vi "PreCompileMainSeq.vi"(6 "steps":i32, 8 "error in (no error)":errorcluster, 9 "first seq":T1, 10 "Compiler Settings":T3={"Python Path"=path "", "Main File"="", "Meta File"="", "Aux File"="", "Pre File"="metascript.txt"}, 11 "queue in":refnum<queue>) -> (0 "error out":errorcluster)   [LabVIEW 2019]
uses:
  PulseCompiler/CompilerSettings.ctl
  Controller/PulseControl.ctl
  Params.ctl
  controls/GlobalExp.vi
  Global.lvlib
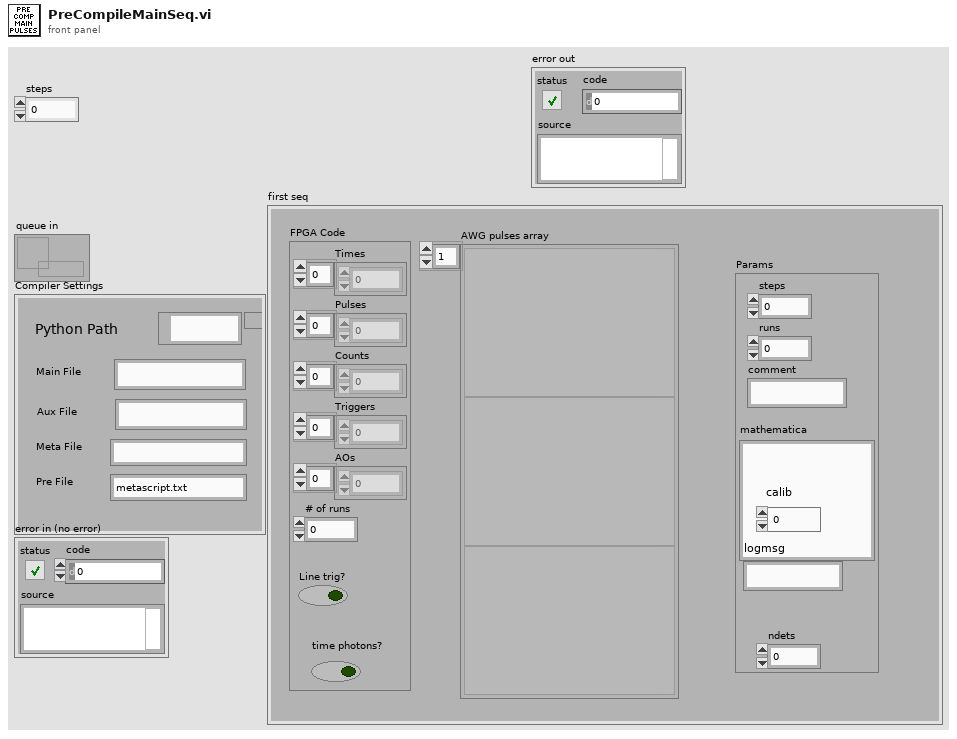
[diagram p1: front panel]
types:
  T1 = typedef "PulseControl.ctl" = cluster{"FPGA Code":cluster{"Times":u32[], "Pulses":u64[], "Counts":u8[], "Triggers":u8[], "AOs":u8[], "# of runs":i32, "Line trig?":bool, "time photons?":bool}, "AWG pulses array":variant[], "Params":T2}
  T2 = typedef "Params.ctl" = cluster{"steps":i16, "runs":i16, "comment":string, "mathematica":string, "calib":i8, "logmsg":string, "ndets":i16}
  T3 = typedef "CompilerSettings.ctl" = cluster{"Python Path":path, "Main File":string, "Meta File":string, "Aux File":string, "Pre File":string}
  T4 = typedef "MasterExpControl.ctl" = cluster{"Main Steps":dbl, "Main Runs":dbl, "ExpStatus":enum16{"Innit", "Stop", "Idle", "MainRunning", "AuxRunning"}, "Main Current Step":dbl, "ExpNum":dbl, "NewData":bool, "date":string, "command":string, "Stop":bool, "Pause":bool, "Mathematica":string, "Main/Meta":bool, "UpdateMath":bool, "Camera":bool, "MetaExpOver":bool, "NextMetaExp":bool}
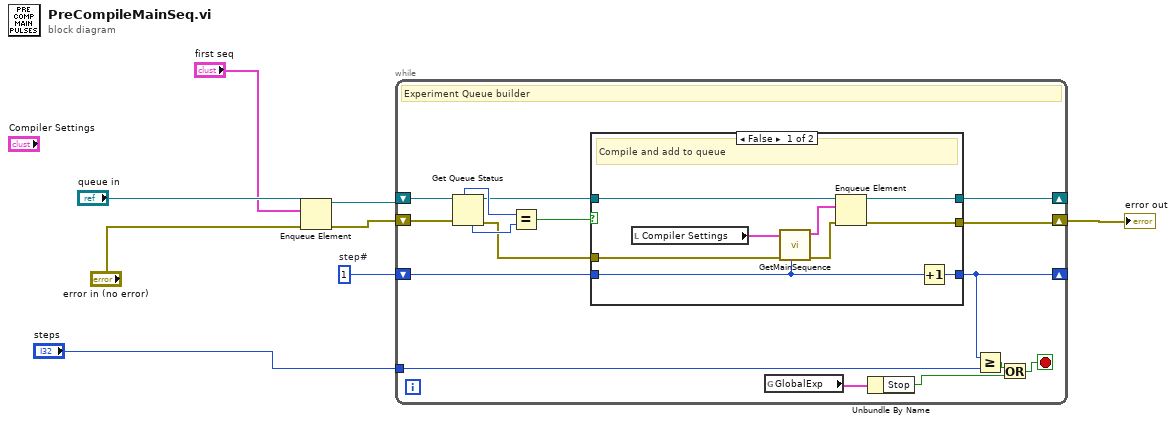
[diagram p0: block diagram]
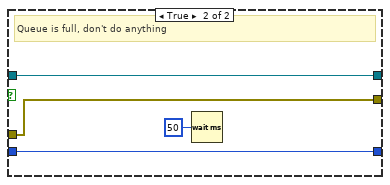
[diagram p2: hidden frame]
diagram:
  w3 = 1  # step#
  n1 = Enqueue Element(queue="queue in", element="first seq", error in (no error)="error in (no error)") -> (queue out=w6:refnum<queue>, error out=w7:errorcluster)  [unwired: 1 in, 1 out]
  n2 = while {
    shift-right: [w18] -> _
    shift-left: w3 -> [w20]
    tunnel: "steps" -> [w19]
    shift-right: [w16] -> _
    shift-left: w6 -> [w24]
    shift-right: [w13] -> w2
    shift-left: w7 -> [w15]
    stop <- w11 stop-if-true
    # "Experiment Queue builder"
    n3 = Get Queue Status(queue=w24, error in (no error)=w15) -> (queue out=w17:refnum<queue>, max queue size=w23:i32, error out=w14:errorcluster, # elements in queue=w22:i32)  [unwired: 1 in, 4 out]
    n4 = Equal?(x=w23, y=w22) -> (x = y?=w21:bool)
    n5 = case shown="False" w21 {
      tunnel: w20 -> [w32 w37]
      tunnel: [w33 w37] -> w18
      tunnel: w17 -> [w31 w36]
      tunnel: [w30 w36] -> w16
      tunnel: w14 -> [w28 w34]
      tunnel: [w26 w34] -> w13
      frame False {
        # "Compile and add to queue"
        n6 = local read "Compiler Settings"() -> (w25:T3)
        n7 = call "GetMainSequence.vi"("Stepnum"=w32, "error in (no error)"=w28, "Compiler Settings"=w25) -> ("error out"=w27:errorcluster, "Main pulse"=w29:T1)  [unwired: 7 in]
        n8 = Enqueue Element(queue=w31, element=w29, error in (no error)=w27) -> (queue out=w30:refnum<queue>, error out=w26:errorcluster)  [unwired: 1 in, 1 out]
        n9 = Increment(x=w32) -> (x+1=w33:i32)
      }
      frame True {
        # "Queue is full, don't do anything"
        n10 = Wait (ms)(milliseconds to wait=u32 50) -> ()  [unwired: 1 out]
      }
    }
    n11 = global read "GlobalExp.vi" "GlobalExp"() -> (w10:T4)
    n12 = Unbundle By Name(w10) -> ("Stop"=w9:bool)
    n13 = Greater Or Equal?(x=w18, y=w19) -> (x >= y?=w12:bool)
    n14 = Or(x=w12, y=w9) -> (x .or. y?=w11:bool)
  }
  "error out" <- w2
